vi "FallSensor.vi"() -> ()   [LabVIEW 2016]
doc: "Desktop application for Fall Sensor (FS) project. Main features:\n- automatic detection of the FS\n- basic communication with FS device \n- hello and reset messages\n- measurement data transfer request\n- processing, displaying and saving obtained data."
uses:
  Requests/RequestType.ctl
  FallSensor/FSState.ctl
  FallSensor/Sample.ctl
  FallSensor/Data.ctl
  FallSensor/DataType.ctl
  FallSensor/FSContext.ctl
  FTDI/COMConfig.ctl
  <vilib>/Instr/_visa.llb/VISA Configure Serial Port (Instr).vi
panel:
  out "GyroData":dbl[][](graph)
  out "AccelData":dbl[][](graph)
  out "Packets":T1[][](array[typedef])
  out "MeasurementFreq[Hz]":u32
  out "DownloadSuccess":bool
  out "AvailablePacket(s)":u32
  out "FallSensorDetected":bool
  out "State":T4
  out "Response":string
  out "LastRequest":T5
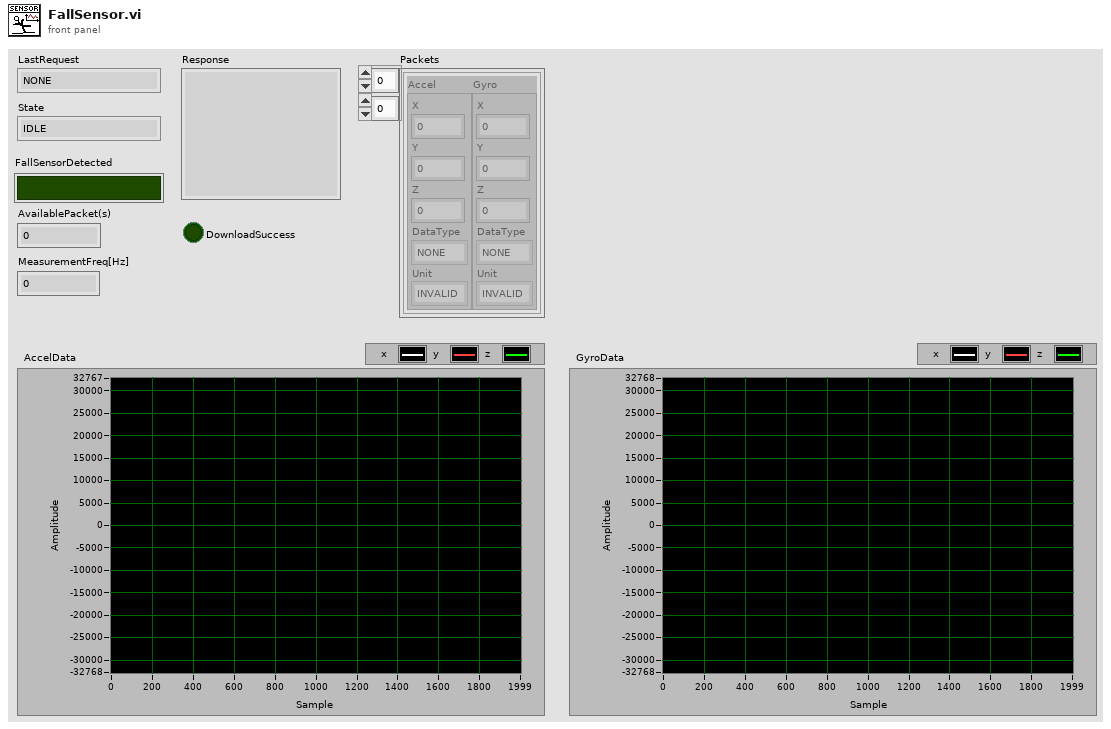
[diagram p1: front panel]
types:
  T1 = typedef "Sample.ctl" = cluster{"Accel":T2, "Gyro":T2}
  T2 = typedef "Data.ctl" = cluster{"X":dbl, "Y":dbl, "Z":dbl, "DataType":T3, "Unit":enum16{"INVALID", "g", "°/sec"}}
  T3 = typedef "DataType.ctl" = enum16{"NONE", "ACCEL", "GYRO"}
  T4 = typedef "FSState.ctl" = enum16{"IDLE", "WaitForEvent", "HandleErrors", "Init", "DetectDevice", "GetAvailablePacketsNr", "EstablishConnection", "CheckPacketsNr", "AskForDataTransfer", "GetMeasurementFrequency", "GetPackets", "DisplayPacket", "Stop"}
  T5 = typedef "RequestType.ctl" = enum16{"NONE", "Reset", "Hello", "GetPacketsNr", "GetMeasFreq", "GetPacket"}
  T6 = typedef "FSContext.ctl" = cluster{"COMHandler":refnum<visa-resource-name>, "COMConfig":T7, "HelloResponse":string, "DeviceDetected":bool, "MeasurementFrequency":u32, "AvailablePacketsNr":u32, "RequestType":T5, "Response":string, "DownloadSuccess":bool, "Packets":T1[][]}
  T7 = typedef "COMConfig.ctl" = cluster{"BaudRate":u32, "DataBits":u16, "Parity":enum16{"None", "Odd", "Even", "Mark", "Space"}, "StopBits":u16, "Timeout[ms]":u32}
  T8 = enum32{"Invalid", "Standard", "Closed", "Hidden", "Minimized", "Maximized"}
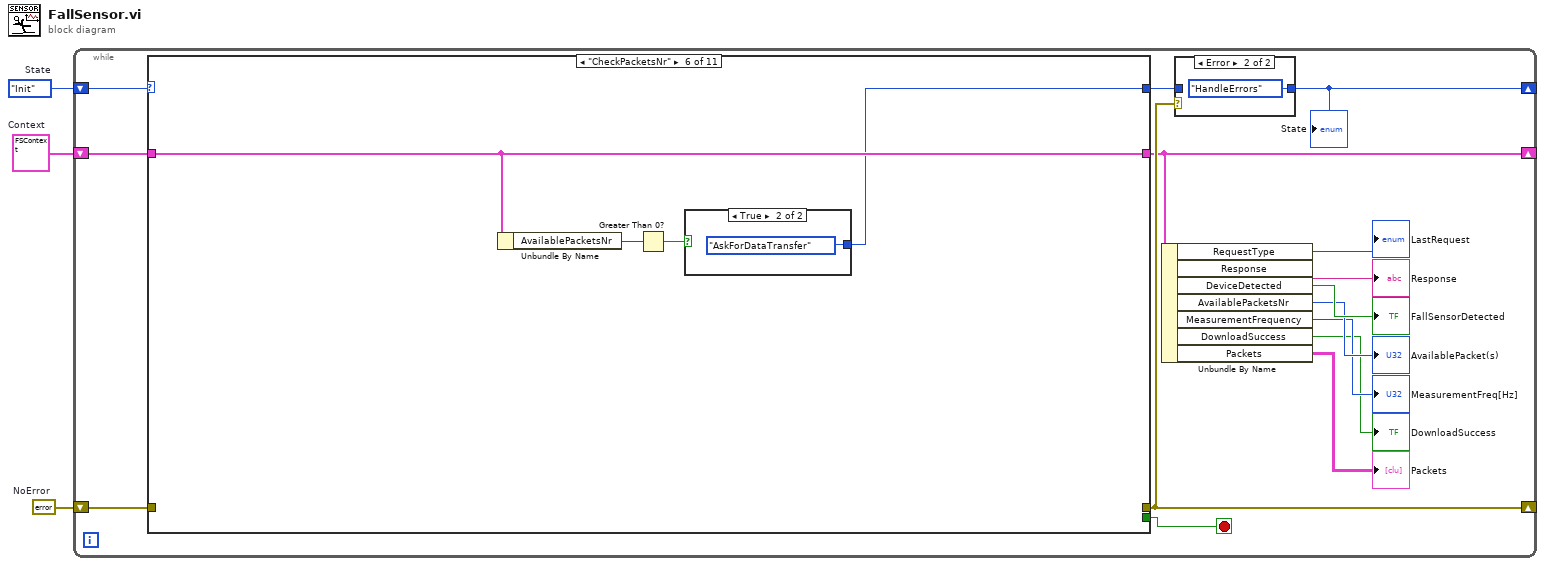
[diagram p0: block diagram]
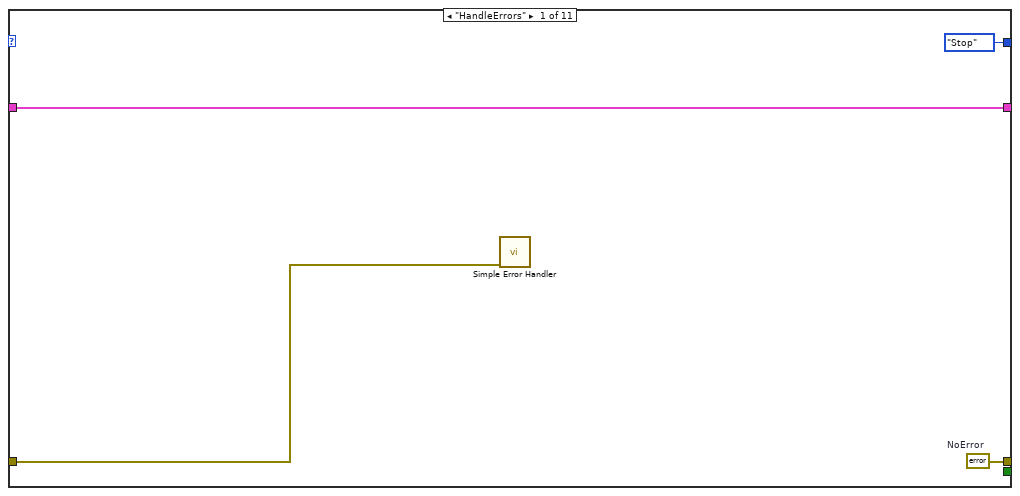
[diagram p2: hidden frame]
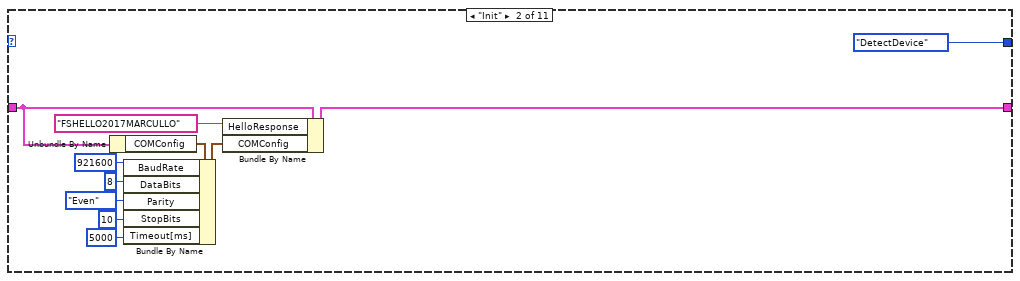
[diagram p3: hidden frame]
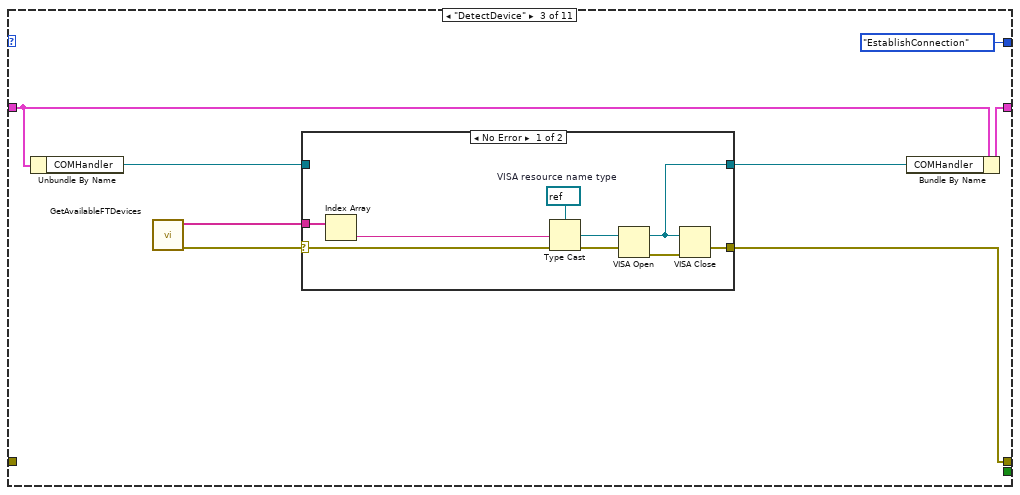
[diagram p4: hidden frame]
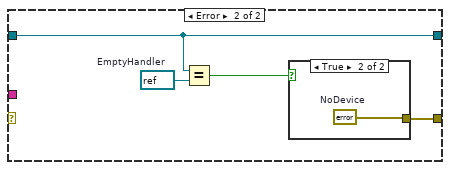
[diagram p5: hidden frame]
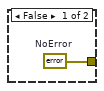
[diagram p6: hidden frame]
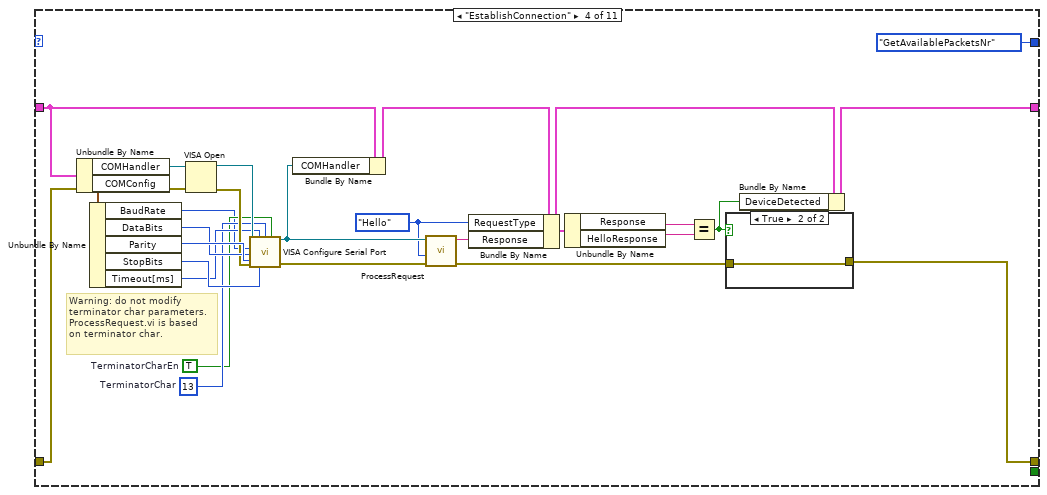
[diagram p7: hidden frame]
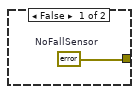
[diagram p8: hidden frame]
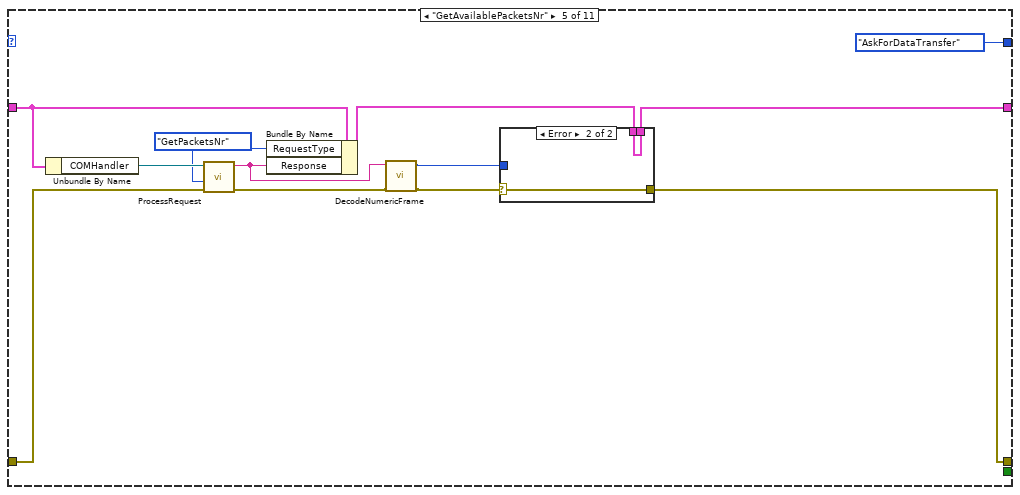
[diagram p9: hidden frame]
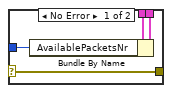
[diagram p10: hidden frame]
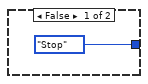
[diagram p11: hidden frame]
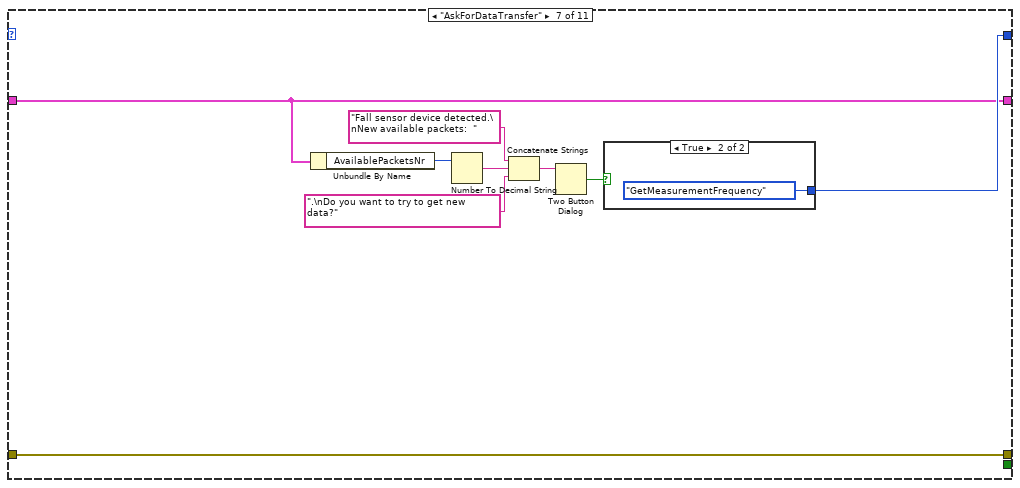
[diagram p12: hidden frame]
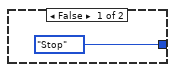
[diagram p13: hidden frame]
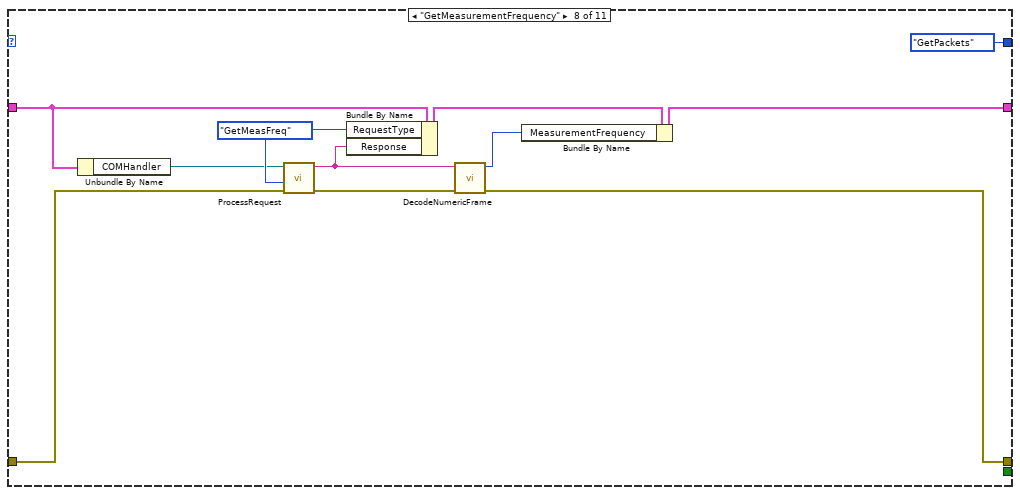
[diagram p14: hidden frame]
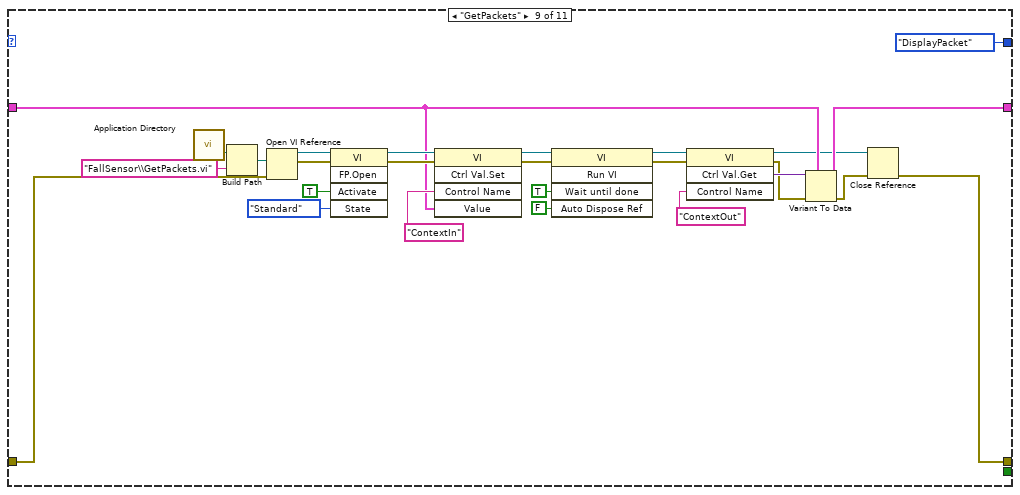
[diagram p15: hidden frame]
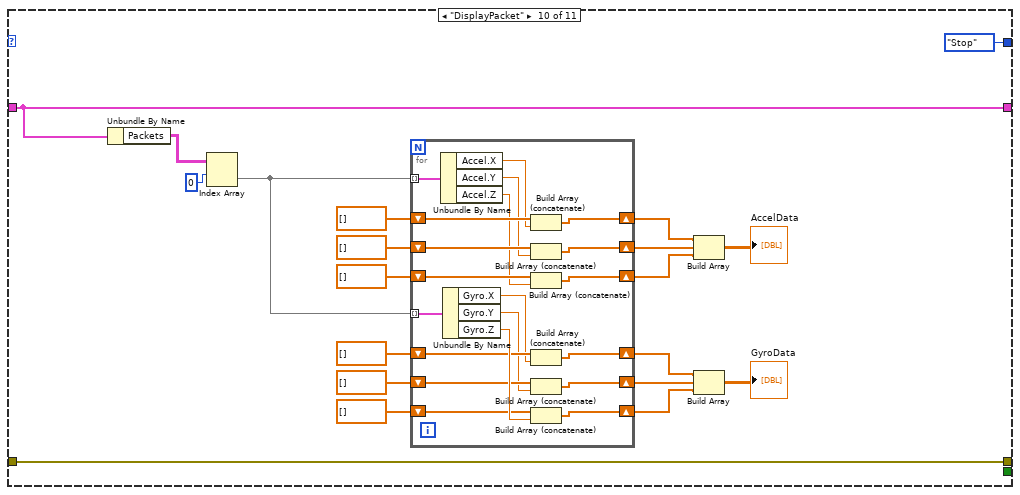
[diagram p16: hidden frame]
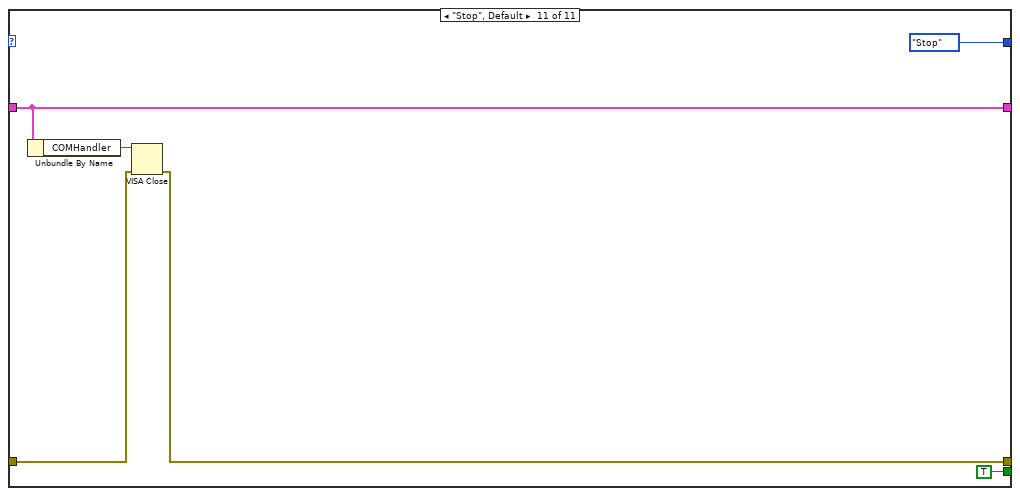
[diagram p17: hidden frame]
diagram:
  w2 = T6 {"COMHandler"="", "COMConfig"={"BaudRate"=9600, "DataBits"=8, "Parity"=enum."None", "StopBits"=10, "Timeout[ms]"=10000}, "HelloResponse"="", "DeviceDetected"=FALSE, "MeasurementFrequency"=0, "AvailablePacketsNr"=0, "RequestType"=enum."NONE", "Response"="", "DownloadSuccess"=FALSE, "Packets"=[]}  # Context
  w3 = errorcluster {"status"=FALSE, "code"=0, "source"=""}  # NoError
  w1 = FSState."Init"  # State
  n1 = while {
    shift-right: [w4] -> _
    shift-left: w1 -> [w5]
    shift-right: [w16] -> _
    shift-left: w3 -> [w18]
    shift-right: [w11] -> _
    shift-left: w2 -> [w17]
    stop <- w15 stop-if-true
    n2 = case shown="\"CheckPacketsNr\"" w5 {
      tunnel: [FSState."Stop" ("State") FSState."DetectDevice" ("State") FSState."EstablishConnection" ("State") FSState."GetAvailablePacketsNr" ("State") FSState."AskForDataTransfer" ("State") w102 w115 FSState."GetPackets" ("State") FSState."DisplayPacket" ("State") FSState."Stop" ("State") FSState."Stop" ("State")] -> w14
      tunnel: [_ _ _ _ _ _ _ _ _ _ TRUE] -> w15
      tunnel: w18 -> [w22 _ _ w74 w91 _ w114 w123 w146 w173 w197]
      tunnel: w17 -> [w19 w26 w37 w73 w93 w103 w108 w119 w135 w174 w199]
      tunnel: [w19 w23 w35 w60 w89 w103 w108 w121 w134 w174 w199] -> w11
      tunnel: [w20 _ w34 w62 w88 _ w114 w122 w139 w173 w196] -> w16
      frame "HandleErrors" {
        w20 = errorcluster {"status"=FALSE, "code"=0, "source"=""}  # NoError
        n3 = call <vilib>:"Simple Error Handler.vi"("error in (no error)"=w22) -> ()  [unwired: 4 in, 5 out]
      }
      frame "Init" {
        n4 = Unbundle By Name(w26) -> ("COMConfig"=w32:T7)
        n5 = Bundle By Name(cluster=w32, "BaudRate"=u32 921600, "DataBits"=u16 8, "Parity"=enum16{"None", "Odd", "Even", "Mark", "Space"}."Even", "StopBits"=u16 10, "Timeout[ms]"=u32 5000) -> (w27:T7)
        n6 = Bundle By Name(cluster=w26, "HelloResponse"="FSHELLO2017MARCULLO", "COMConfig"=w27) -> (w23:T6)
      }
      frame "DetectDevice" {
        n7 = Unbundle By Name(w37) -> ("COMHandler"=w38:refnum<visa-resource-name>)
        n8 = call "GetAvailableFTDevices.vi"() -> ("ErrorOut"=w40:errorcluster, "COMs"=w39:string[])  [unwired: 8 in, 2 out]
        n9 = case shown="No Error" w40 {
          selector: w40 -> [w45 _]
          tunnel: [w43 w50] -> w34
          tunnel: w39 -> [w49 _]
          tunnel: w38 -> [_ w53]
          tunnel: [w42 w53] -> w36
          frame No Error {
            w47 = refnum<visa-resource-name> refnum  # VISA resource name type
            n10 = Index Array(array=w49) -> (element=w48:string)  [unwired: 1 in]
            n11 = Type Cast(type=w47, x=w48) -> (*(type *) &x=w46:refnum<visa-resource-name>)
            n12 = VISA Open(error in (no error)=w45, VISA resource name=w46) -> (VISA resource name=w42:refnum<visa-resource-name>, error out=w44:errorcluster)  [unwired: 3 in]
            n13 = VISA Close(VISA resource name=w42, error in (no error)=w44) -> (error out=w43:errorcluster)
          }
          frame Error {
            w52 = refnum<visa-resource-name> refnum  # EmptyHandler
            n14 = Equal?(x=w53, y=w52) -> (x = y?=w51:bool)
            n15 = case shown="True" w51 {
              tunnel: [w54 w55] -> w50
              frame False {
                w54 = errorcluster {"status"=FALSE, "code"=0, "source"=""}  # NoError
              }
              frame True {
                w55 = errorcluster {"status"=TRUE, "code"=7, "source"="Device disconnected"}  # NoDevice
              }
            }
          }
        }
        n16 = Bundle By Name(cluster=w37, "COMHandler"=w36) -> (w35:T6)
      }
      frame "EstablishConnection" {
        w65 = RequestType."Hello" ("RequestType")
        w69 = TRUE  # TerminatorCharEn
        w70 = u8 13  # TerminatorChar
        # "Warning: do not modify \nterminator char parameters.\nProcessRequest.vi is based\non terminator char."
        n17 = Unbundle By Name(w73) -> ("COMHandler"=w75:refnum<visa-resource-name>, "COMConfig"=w76:T7)
        n18 = Unbundle By Name(w76) -> ("BaudRate"=w58:u32, "DataBits"=w79:u16, "Parity"=w80:enum16{"None", "Odd", "Even", "Mark", "Space"}, "StopBits"=w81:u16, "Timeout[ms]"=w71:u32)
        n19 = VISA Open(error in (no error)=w74, VISA resource name=w75) -> (VISA resource name=w78:refnum<visa-resource-name>, error out=w77:errorcluster)  [unwired: 3 in]
        n20 = call-poly "VISA Configure Serial Port"("VISA resource name"=w78, "timeout (10sec)"=w71, "termination char\n(0xA = '\\n' = LF)"=w70, "Enable Termination\nChar (T)"=w69, "baud rate (9600)"=w58, "data bits (8)"=w79, "parity (0:none)"=w80, "error in (no error)"=w77, "stop bits (10: 1 bit)"=w81) -> ("VISA resource name out"=w66:refnum<visa-resource-name>, "error out"=w68:errorcluster)  [unwired: 5 in]
        n21 = Bundle By Name(cluster=w73, "COMHandler"=w66) -> (w67:T6)
        n22 = call "ProcessRequest.vi"("ErrorIn"=w68, "RequestType"=w65, "DeviceResourceName"=w66) -> ("ErrorOut"=w63:errorcluster, "Response"=w64:string)  [unwired: 5 in, 2 out]
        n23 = Bundle By Name(cluster=w67, "RequestType"=w65, "Response"=w64) -> (w61:T6)
        n24 = Unbundle By Name(w61) -> ("Response"=w56:string, "HelloResponse"=w57:string)
        n25 = Equal?(x=w56, y=w57) -> (x = y?=w59:bool)
        n26 = case shown="True" w59 {
          tunnel: w63 -> [_ w83]
          tunnel: [w82 w83] -> w62
          frame False {
            w82 = errorcluster {"status"=TRUE, "code"=8, "source"="Fall Sensor not recognized"}  # NoFallSensor
          }
          frame True {
          }
        }
        n27 = Bundle By Name(cluster=w61, "DeviceDetected"=w59) -> (w60:T6)
      }
      frame "GetAvailablePacketsNr" {
        w92 = RequestType."GetPacketsNr" ("RequestType")
        n28 = Unbundle By Name(w93) -> ("COMHandler"=w94:refnum<visa-resource-name>)
        n29 = call "ProcessRequest.vi"("ErrorIn"=w91, "RequestType"=w92, "DeviceResourceName"=w94) -> ("ErrorOut"=w85:errorcluster, "Response"=w87:string)  [unwired: 5 in, 2 out]
        n30 = Bundle By Name(cluster=w93, "RequestType"=w92, "Response"=w87) -> (w90:T6)
        n31 = call "DecodeNumericFrame.vi"("ErrorIn"=w85, "Frame"=w87) -> ("ErrorOut"=w84:errorcluster, "ReceivedValue"=w86:u32)  [unwired: 8 in]
        n32 = case shown="Error" w84 {
          selector: w84 -> [w96 w100]
          tunnel: w86 -> [w99 _]
          tunnel: w90 -> [w98 w101]
          tunnel: [w97 w101] -> w89
          tunnel: [w96 w100] -> w88
          frame No Error {
            n33 = Bundle By Name(cluster=w98, "AvailablePacketsNr"=w99) -> (w97:T6)
          }
          frame Error {
          }
        }
      }
      frame "CheckPacketsNr" {
        n34 = Unbundle By Name(w103) -> ("AvailablePacketsNr"=w105:u32)
        n35 = Greater Than 0?(x=w105) -> (x > 0?=w104:bool)
        n36 = case shown="True" w104 {
          tunnel: [FSState."Stop" ("State") FSState."AskForDataTransfer" ("State")] -> w102
          frame False {
          }
          frame True {
          }
        }
      }
      frame "AskForDataTransfer" {
        n37 = Unbundle By Name(w108) -> ("AvailablePacketsNr"=w110:u32)
        n38 = Number To Decimal String(number=w110) -> (decimal integer string=w109:string)  [unwired: 1 in]
        n39 = Concatenate Strings("Fall sensor device detected.\nNew available packets:  " ("message"), w109, ".\nDo you want to try to get new data?" ("string")) -> (w111:string)
        n40 = Two Button Dialog(message=w111) -> (T button?=w116:bool)  [unwired: 2 in]
        n41 = case shown="True" w116 {
          tunnel: [FSState."Stop" ("State") FSState."GetMeasurementFrequency" ("State")] -> w115
          frame False {
          }
          frame True {
          }
        }
      }
      frame "GetMeasurementFrequency" {
        w129 = RequestType."GetMeasFreq" ("RequestType")
        n42 = Unbundle By Name(w119) -> ("COMHandler"=w128:refnum<visa-resource-name>)
        n43 = call "ProcessRequest.vi"("ErrorIn"=w123, "RequestType"=w129, "DeviceResourceName"=w128) -> ("ErrorOut"=w125:errorcluster, "Response"=w126:string)  [unwired: 5 in, 2 out]
        n44 = Bundle By Name(cluster=w119, "RequestType"=w129, "Response"=w126) -> (w127:T6)
        n45 = call "DecodeNumericFrame.vi"("ErrorIn"=w125, "Frame"=w126) -> ("ErrorOut"=w122:errorcluster, "ReceivedValue"=w124:u32)  [unwired: 8 in]
        n46 = Bundle By Name(cluster=w127, "MeasurementFrequency"=w124) -> (w121:T6)
      }
      frame "GetPackets" {
        n47 = call <vilib>:"Application Directory.vi"() -> ("Application Directory"=w148:path)
        n48 = Build Path(base path=w148, name or relative path="FallSensor\\GetPackets.vi") -> (appended path=w147:path)
        n49 = Open VI Reference(vi path=w147, error in (no error)=w146) -> (vi reference=w145:refnum<vi>, error out=w144:errorcluster)  [unwired: 4 in]
        n50 = invoke class="VI" method="FP.Open"(reference=w145, error in=w144, "Activate"=TRUE ("Activate?"), "State"=T8."Standard") -> (reference out=w150:refnum<vi>, error out=w143:errorcluster)  [unwired: 1 in, 3 out]
        n51 = invoke class="VI" method="Ctrl Val.Set"(reference=w150, error in=w143, "Control Name"="ContextIn", "Value"=w135) -> (reference out=w142:refnum<vi>, error out=w141:errorcluster)  [unwired: 1 in, 3 out]
        n52 = invoke class="VI" method="Run VI"(reference=w142, error in=w141, "Wait until done"=TRUE ("Wait Until Done"), "Auto Dispose Ref"=FALSE ("Auto Dispose Reference")) -> (reference out=w131:refnum<vi>, error out=w130:errorcluster)  [unwired: 1 in, 3 out]
        n53 = invoke class="VI" method="Ctrl Val.Get"(reference=w131, error in=w130, "Control Name"="ContextOut") -> (reference out=w133:refnum<vi>, error out=w136:errorcluster, "Get Control Value Variant"=w137:variant)  [unwired: 1 in, 1 out]
        n54 = Variant To Data(error in=w136, type=w135, Variant=w137) -> (data=w134:T6, error out=w132:errorcluster)
        n55 = Close Reference(reference=w133, error in (no error)=w132) -> (error out=w139:errorcluster)
      }
      frame "DisplayPacket" {
        n56 = Unbundle By Name(w174) -> ("Packets"=w172:T1[][])
        n57 = Index Array(array=w172, index (row)=0 ("disabled index (col)")) -> (element=w157:T1[])  [unwired: 1 in]
        n58 = for {
          tunnel: w157 -> [w194] mode=indexing
          shift-right: [w192] -> w167
          shift-left: dbl[] [] -> [w195]
          shift-right: [w187] -> w168
          shift-left: dbl[] [] -> [w191]
          shift-right: [w186] -> w166
          shift-left: dbl[] [] -> [w190]
          shift-right: [w180] -> w162
          shift-left: dbl[] [] -> [w179]
          shift-right: [w184] -> w161
          shift-left: dbl[] [] -> [w181]
          shift-right: [w185] -> w163
          shift-left: dbl[] [] -> [w182]
          tunnel: w157 -> [w178] mode=indexing
          n59 = Unbundle By Name(w194) -> ("Accel.X"=w193:dbl, "Accel.Y"=w189:dbl, "Accel.Z"=w188:dbl)
          n60 = Unbundle By Name(w178) -> ("Gyro.X"=w177:dbl, "Gyro.Y"=w176:dbl, "Gyro.Z"=w183:dbl)
          n61 = Build Array (concatenate)(w195, w193) -> (w192:dbl[])
          n62 = Build Array (concatenate)(w191, w189) -> (w187:dbl[])
          n63 = Build Array (concatenate)(w190, w188) -> (w186:dbl[])
          n64 = Build Array (concatenate)(w179, w177) -> (w180:dbl[])
          n65 = Build Array (concatenate)(w181, w176) -> (w184:dbl[])
          n66 = Build Array (concatenate)(w182, w183) -> (w185:dbl[])
        }
        n67 = Build Array(w167, w168, w166) -> (→"AccelData":dbl[][])
        n68 = Build Array(w162, w161, w163) -> (→"GyroData":dbl[][])
      }
      frame "Stop", Default {
        n69 = Unbundle By Name(w199) -> ("COMHandler"=w198:refnum<visa-resource-name>)
        n70 = VISA Close(VISA resource name=w198, error in (no error)=w197) -> (error out=w196:errorcluster)
      }
    }
    n71 = Unbundle By Name(w11) -> ("RequestType"=→"LastRequest":T5, "Response"=→"Response":string, "DeviceDetected"=→"FallSensorDetected":bool, "AvailablePacketsNr"=→"AvailablePacket(s)":u32, "MeasurementFrequency"=→"MeasurementFreq[Hz]":u32, "DownloadSuccess"=→"DownloadSuccess":bool, "Packets"=→"Packets":T1[][])
    n72 = case shown="Error" w16 {
      tunnel: w14 -> [w202 _]
      tunnel: [w202 FSState."HandleErrors" ("State")] -> w4
      frame No Error {
      }
      frame Error {
      }
    }
    "State" <- w4
  }
